vi "Taiko_UIntToPrefix.vi"(11 "UINT":u32) -> (2 "PREFIX":string, 3 "MANT":sgl)   [LabVIEW 2010]
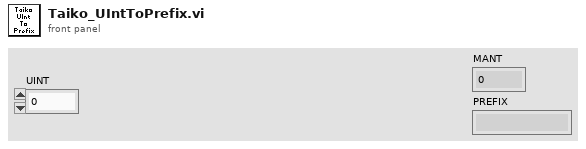
[diagram p1: front panel]
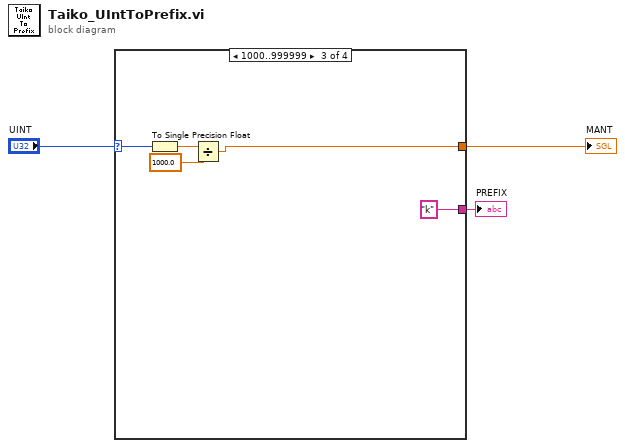
[diagram p0: block diagram]
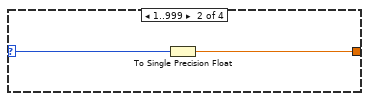
[diagram p3: hidden frame]
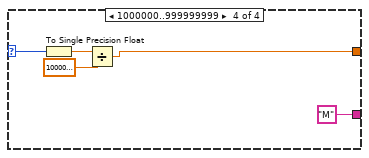
[diagram p4: hidden frame]
diagram:
  n1 = case shown="1000..999999" "UINT" {
    selector: "UINT" -> [w4 w6 w10 w15]
    tunnel: [w4 w5 w8 w13] -> w2
    tunnel: [_ _ "k" "M"] -> w1
    frame Default {
    }
    frame 1..999 {
      n2 = To Single Precision Float(number=w6) -> (single precision float=w5:sgl)
    }
    frame 1000..999999 {
      n3 = To Single Precision Float(number=w10) -> (single precision float=w9:sgl)
      n4 = Divide(x=w9, y=sgl 1000.0) -> (x/y=w8:sgl)
    }
    frame 1000000..999999999 {
      n5 = To Single Precision Float(number=w15) -> (single precision float=w14:sgl)
      n6 = Divide(x=w14, y=sgl 1000000.0) -> (x/y=w13:sgl)
    }
  }
  "MANT" <- w2
  "PREFIX" <- w1
